vi "XPath File Sub-Parser.vi"(3 "error in (no error)":errorcluster, 4 "XPath Expression":string, 5 "XML File Path In":path) -> (0 "error out":errorcluster, 1 "Array of Results":string[](array[string]), 2 "XML File Path Out":path)   [LabVIEW 2013]
doc: "Use an XPath expression to search an XML file. An array containing all instances matching the search criteria will be returned."
uses:
  <vilib>/xml/Close Reference(Node).vi
  <vilib>/xml/NI_XML.lvlib
  <resource>/objmgr/DOMUserDefRef.rc
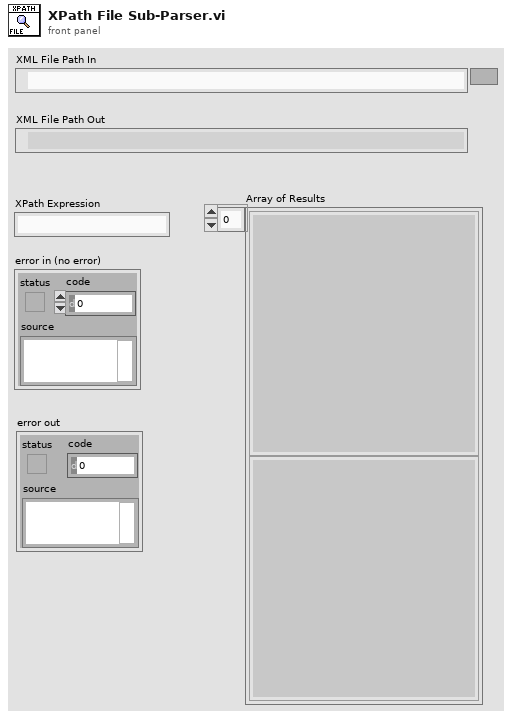
[diagram p1: front panel]
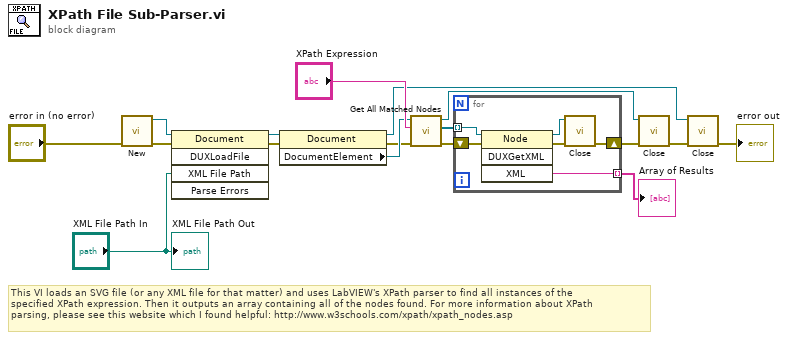
[diagram p0: block diagram]
diagram:
  # "This VI loads an SVG file (or any XML file for that matter) and uses LabVIEW's XPath parser to find all instances of the\nspecified XPath expression. Then it outputs an array containing all of the nodes found. For more information about XPath\nparsing, please see this website which I found helpful: http://www.w3schools.com/xpath/xpath_nodes.asp"
  n1 = call <vilib>:"New.vi"("error in (no error)"="error in (no error)") -> ("error out"=w16:errorcluster, "DOM document out"=w12:refnum<k20>)  [unwired: 7 in]
  n2 = invoke class="Document" method="DUXLoadFile"(reference=w12, error in=w16, "XML File Path"="XML File Path In") -> (reference out=w14:refnum<k20>, error out=w15:errorcluster)  [unwired: 2 in, 3 out]
  n3 = property class="Document"(reference=w14, error in=w15) -> (reference out=w2:refnum<k20>, error out=w6:errorcluster, "DocumentElement"=w8:refnum<k20>)
  n4 = call <vilib>:"Get All Matched Nodes.vi"("error in (no error)"=w6, "XPath expression"="XPath Expression", "node in"=w8) -> ("error out"=w7:errorcluster, "node result array"=w5:refnum<k20>[], "node out"=w1:refnum<k20>)  [unwired: 6 in]
  n5 = for {
    tunnel: w5 -> [w23] mode=indexing
    tunnel: [w22] -> w9 mode=indexing
    shift-right: [w18] -> w4
    shift-left: w7 -> [w21]
    n6 = invoke class="Node" method="DUXGetXML"(reference=w23, error in=w21) -> (reference out=w20:refnum<k20>, error out=w19:errorcluster, "XML"=w22:string)  [unwired: 2 in, 1 out]
    n7 = call-poly <vilib>:"Close.vi"("error in (no error)"=w19, "node"=w20) -> ("error out"=w18:errorcluster)  [unwired: 7 in]
  }
  "Array of Results" <- w9
  n8 = call-poly <vilib>:"Close.vi"("error in (no error)"=w4, "node"=w1) -> ("error out"=w3:errorcluster)  [unwired: 7 in]
  n9 = call-poly <vilib>:"Close.vi"("error in (no error)"=w3, "node"=w2) -> ("error out"=→"error out":errorcluster)  [unwired: 7 in]
  "XML File Path Out" <- "XML File Path In"
